vi "LCOS GUI v3_green.vi"() -> ()   [LabVIEW 2011]
uses:
  Periodic Spot Pattern Parameters.ctl
  LCOS State Machine States.ctl
  LCOS Pattern Display Actions.ctl
  LCOS Parent Action.ctl
  LCOS Images.ctl
  <vilib>/vision/Image Controls.llb/IMAQ Image.ctl
panel:
  in  "Enable Remote Control":bool=TRUE
  in  "Clear Error":bool
  in  "Ignore":bool
  out "Last Error":errorcluster
  in  "Loaded Pattern File:":bool
  out "File Path":path
  out "LCOS Pattern Preview":T1(plugin-control)
  in  "Buttons":T2={"Pattern"=enum."Computed", "Auto-Update LCOS"=TRUE, "Apply Correction"=FALSE, "Update LCOS"=FALSE, "Preview Pattern"=FALSE, "Auto-Preview"=TRUE}
  in  "Pattern Definition":T3={"X pitch"=24.0, "rotation"=0.0, "Center H"=0.0, "Center V"=0.0, "# Spots H"=4, "# Spots V"=12, "Spot size"=20.0, "ref_spot _dark"=FALSE, "Exact Phase Formula"=FALSE, "phase_wrap_pos"=FALSE, "Set Focus (mm)"=36.0, "phase_max"=3.0, "phase_factor"=82, "Steer LW"=1, "Steer vmax"=95, "phase_wrap_neg"=TRUE, "steer_horiz"=TRUE, "steer_pad"=10, "steer_only"=FALSE, "Wavelength"=5.32e-07, "Y pitch"=24.0, "python"=TRUE, "test_pattern"=FALSE, "grid"=TRUE, "dark_all"=FALSE, "Xm_str"="", "Ym_str"="", "ref_spot"=6, "stretch"=FALSE} {"ref_spot" min=0 max=500 step=1 format="%#.0f"; "Y pitch" min=0.0 max=100.0 format="%.2g"; "Wavelength" min=0.0 max=500.0 format="%^#.3e"; "steer_pad" min=0 max=500 step=1 format="%#.0f"; "Steer LW" max=500; "phase_max" min=0.0 max=500.0 format="%#.3f"; "Set Focus (mm)" min=0.0 max=500.0 format="%#.3g"; "Spot size" min=1.0 format="%.2g"; "# Spots V" min=1 step=1; "# Spots H" min=1 step=1; "Center V" format="%.2f"; "Center H" format="%.2f"; "rotation" min=-90.0 max=90.0 format="%.2g"; "X pitch" min=0.0 max=100.0 format="%.2g"}
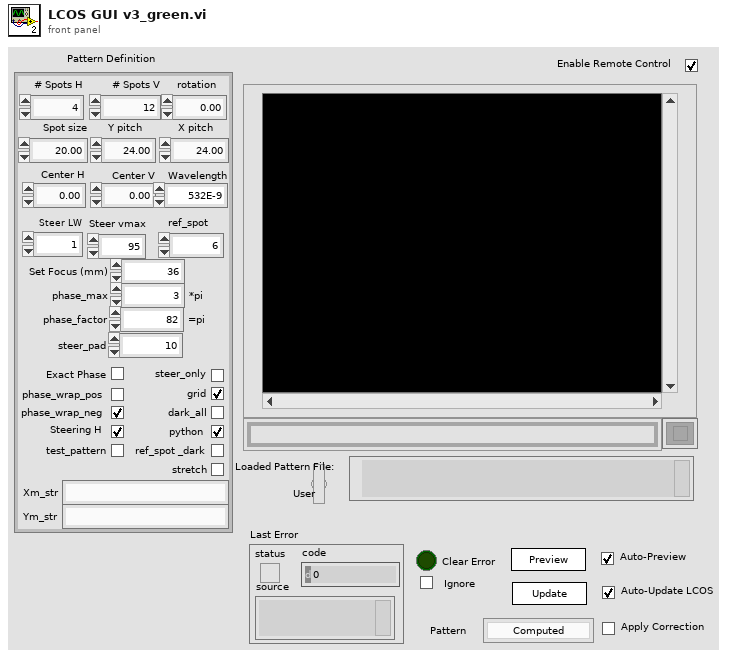
[diagram p1: front panel]
types:
  T1 = typedef "IMAQ Image.ctl" = refnum<image>
  T2 = cluster{"Pattern":enum16{"Computed", "From File", "Correction"}, "Auto-Update LCOS":bool, "Apply Correction":bool, "Update LCOS":bool, "Preview Pattern":bool, "Auto-Preview":bool}
  T3 = typedef "Periodic Spot Pattern Parameters.ctl" = cluster{"X pitch":dbl, "rotation":dbl, "Center H":dbl, "Center V":dbl, "# Spots H":u32, "# Spots V":u32, "Spot size":dbl, "ref_spot _dark":bool, "Exact Phase Formula":bool, "phase_wrap_pos":bool, "Set Focus (mm)":dbl, "phase_max":dbl, "phase_factor":u8, "Steer LW":u32, "Steer vmax":u8, "phase_wrap_neg":bool, "steer_horiz":bool, "steer_pad":i64, "steer_only":bool, "Wavelength":dbl, "Y pitch":dbl, "python":bool, "test_pattern":bool, "grid":bool, "dark_all":bool, "Xm_str":string, "Ym_str":string, "ref_spot":i64, "stretch":bool}
  T4 = typedef "LCOS Pattern Display Actions.ctl" = enum16{"Init", "Idle", "Update", "Exit"}
  T5 = cluster{"LCOS Pattern Display Actions":T4, "Data":variant}
  T6 = typedef "LCOS State Machine States.ctl" = enum16{"Init", "Idle", "Preview Button Pushed", "Update Button Pushed", "Pattern Selection Changed", "Pattern Definition Changed", "Selected File Changed", "Load Correction Pattern", "Load Correction Pattern Step 2", "Load User Pattern", "Load User Pattern Step 2", "Compute Pattern", "Correct Pattern", "Update Preview Display", "Update LCOS Display", "Error", "Clear Error", "Exit"}
  T7 = cluster{"X pitch":dbl, "rotation":dbl, "Center H":dbl, "Center V":dbl, "# Spots H":u32, "# Spots V":u32, "Spot size":dbl, "ref_spot _dark":bool, "Exact Phase Formula":bool, "phase_wrap_pos":bool, "Set Focus (mm)":dbl, "phase_max":dbl, "phase_factor":u8, "Steer LW":u32, "Steer vmax":u8, "phase_wrap_neg":bool, "steer_horiz":bool, "steer_pad":i64, "steer_only":bool, "Wavelength":dbl, "Y pitch":dbl, "python":bool, "test_pattern":bool, "grid":bool, "dark_all":bool, "Xm_str":string, "Ym_str":string, "ref_spot":i64, "stretch":bool}
  T8 = typedef "LCOS Parent Action.ctl" = enum16{"Pattern Definition Changed", "Preview Button Pushed", "Update Button Pushed", "Pattern Selection Changed", "Correction Pattern Changed", "User Pattern (from File) Changed"}
  T9 = typedef "LCOS Images.ctl" = cluster{"Computed Pattern Image":T1, "User Pattern (from File) Image":T1, "Correction Pattern Image":T1, "Corrected Pattern Image":T1, "Preview Image":T1, "LCOS Displayed Image":T1}
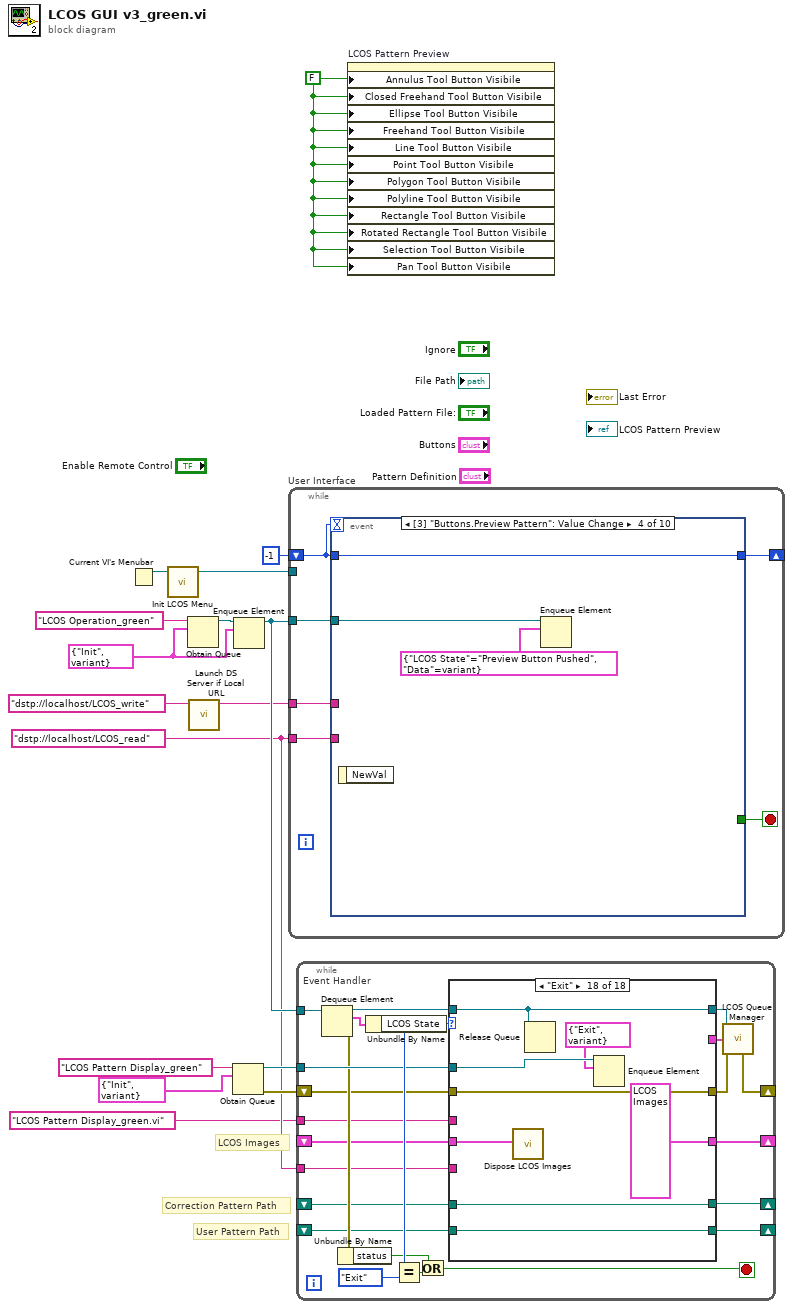
[diagram p0: block diagram]
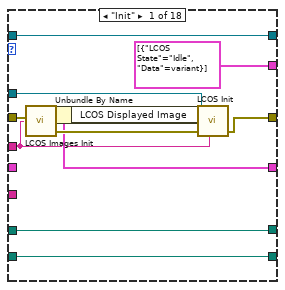
[diagram p2: hidden frame]
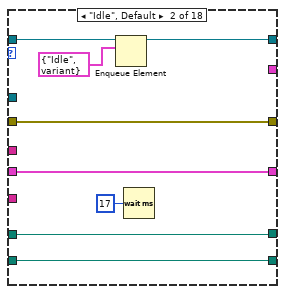
[diagram p3: hidden frame]
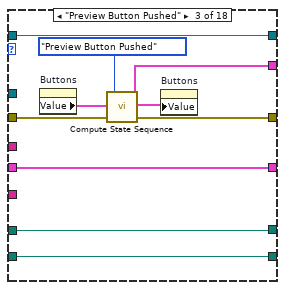
[diagram p4: hidden frame]
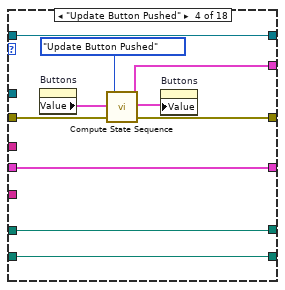
[diagram p5: hidden frame]
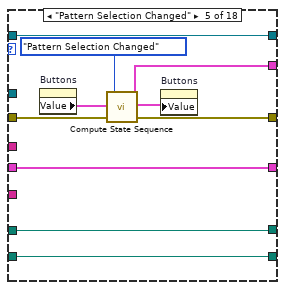
[diagram p6: hidden frame]
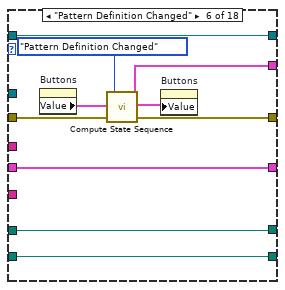
[diagram p7: hidden frame]
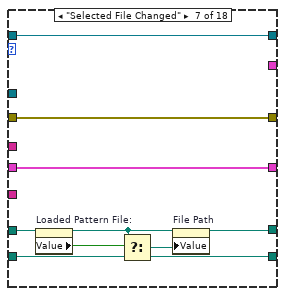
[diagram p8: hidden frame]
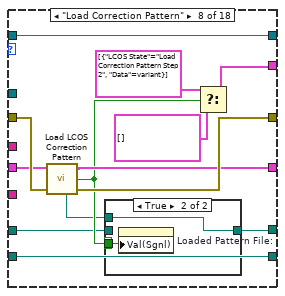
[diagram p9: hidden frame]
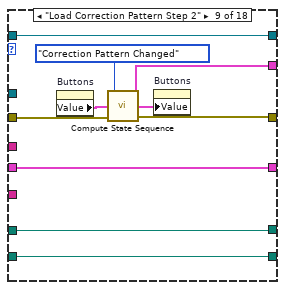
[diagram p11: hidden frame]
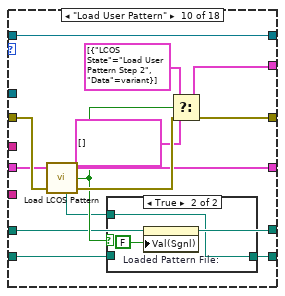
[diagram p12: hidden frame]
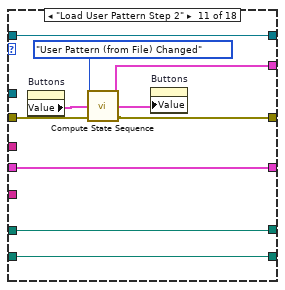
[diagram p14: hidden frame]
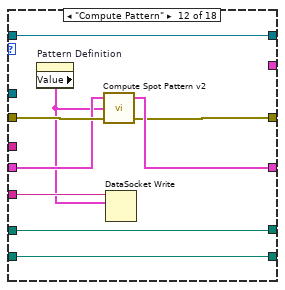
[diagram p15: hidden frame]
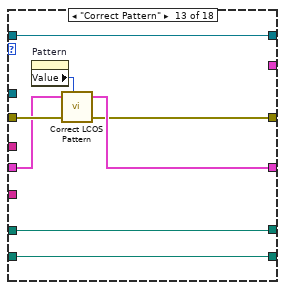
[diagram p16: hidden frame]
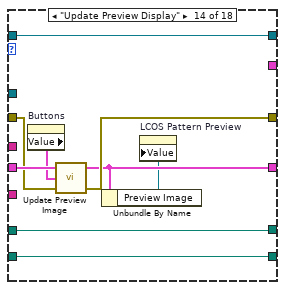
[diagram p17: hidden frame]
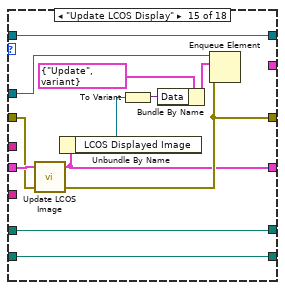
[diagram p18: hidden frame]
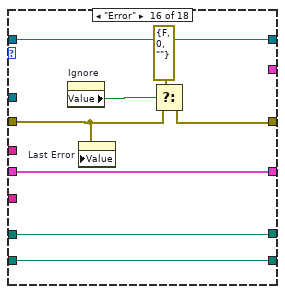
[diagram p19: hidden frame]
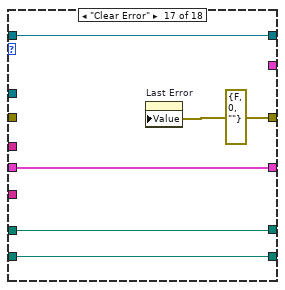
[diagram p20: hidden frame]
diagram:
  w2 = "dstp://localhost/LCOS_read" ("URL")
  w6 = FALSE ("ROI Tool Buttons Visibile:Annulus Tool Button Visibile")
  w7 = cluster{"LCOS State":T6, "Data":variant} {"LCOS State"=enum."Init", "Data"=variant}
  # "User Pattern Path"
  # "Correction Pattern Path"
  # "LCOS Images"
  n1 = Current VI's Menubar() -> (w16:refnum<k9>)
  n2 = call "Init LCOS Menu.vi"("Menu Refnum (in)"=w16) -> ("Menu Refnum (out)"=w15:refnum<k9>)  [unwired: 7 in, 1 out]
  n3 = Obtain Queue(name (unnamed)="LCOS Operation_green", element data type=w7) -> (queue out=w9:refnum<queue>)  [unwired: 3 in, 2 out]
  n4 = call "Launch DS Server if Local URL.vi"("URL"="dstp://localhost/LCOS_write") -> ("Duplicate URL"=w3:string)  [unwired: 5 in, 1 out]
  n5 = Obtain Queue(name (unnamed)="LCOS Pattern Display_green", element data type=T5 {"LCOS Pattern Display Actions"=enum."Init", "Data"=variant}) -> (queue out=w11:refnum<queue>, error out=w10:errorcluster)  [unwired: 3 in, 1 out]
  n6 = Enqueue Element(queue=w9, element=w7) -> (queue out=w8:refnum<queue>)  [unwired: 2 in, 2 out]
  n7 = while "User Interface" {
    tunnel: w15 -> [_]
    tunnel: w8 -> [w21]
    shift-right: [w20] -> _
    shift-left: -1 -> [w19]
    tunnel: w3 -> [w18]
    tunnel: w2 -> [w17]
    stop <- w22 stop-if-true
    n8 = event shown="[3] \"Buttons.Preview Pattern\": Value Change" {
      selector: _ -> [_ _ _ _ _ _ _ _ _ _]
      dyn-events: _ -> [_ _ _ _ _ _ _ _ _ _]
      timeout: w19 -> [_ _ _ _ _ _ _ _ _ _]
      tunnel: [_ _ _ _ _ _ _ _ w58 w76] -> w22
      tunnel: w21 -> [_ _ w41 w44 w47 w50 w53 w56 w59 w75]
      tunnel: [w23 w35 w39 w42 w45 w48 w51 w54 w57 w73] -> w20
      tunnel: w19 -> [w23 _ w39 w42 w45 w48 w51 w54 w57 w73]
      tunnel: w18 -> [w28 _ _ _ _ _ _ _ _ _]
      tunnel: w17 -> [w24 w32 _ _ _ _ _ _ _ _]
      event Timeout {
        n9 = event-data() -> ()  [unwired: 1 in, 1 out]
        n10 = DataSocket Read(9:w23, 10:T3 {"X pitch"=0.0, "rotation"=0.0, "Center H"=0.0, "Center V"=0.0, "# Spots H"=0, "# Spots V"=0, "Spot size"=0.0, "ref_spot _dark"=FALSE, "Exact Phase Formula"=FALSE, "phase_wrap_pos"=FALSE, "Set Focus (mm)"=0.0, "phase_max"=0.0, "phase_factor"=0, "Steer LW"=0, "Steer vmax"=0, "phase_wrap_neg"=FALSE, "steer_horiz"=FALSE, "steer_pad"=0, "steer_only"=FALSE, "Wavelength"=0.0, "Y pitch"=0.0, "python"=FALSE, "test_pattern"=FALSE, "grid"=FALSE, "dark_all"=FALSE, "Xm_str"="", "Ym_str"="", "ref_spot"=0, "stretch"=FALSE} ("Pattern Definition"), 11:w28) -> (1:w26:bool, 2:w25:T3)  [unwired: 2 in, 5 out]
        n11 = case shown="False" w26 {
          tunnel: w25 -> [w30 _]
          tunnel: w24 -> [w31 _]
          tunnel: w23 -> [w29 _]
          frame False {
            n12 = property on="Pattern Definition" class="Clust (strict)"("Val(Sgnl)"=w30) -> ()  [unwired: 2 in, 2 out]
            n13 = DataSocket Write(9:w29, 10:w30, 11:w31) -> ()  [unwired: 1 in, 3 out]
          }
          frame True {
          }
        }
      }
      event "Enable Remote Control": Value Change {
        n14 = event-data() -> ("NewVal"=w33:bool)  [unwired: 1 in]
        n15 = case shown="False" w33 {
          tunnel: w32 -> [_ w38]
          frame False {
          }
          frame True {
            n16 = property on="Pattern Definition" class="Clust (strict)"() -> ("Value"=w37:T7)  [unwired: 2 in, 2 out]
            n17 = DataSocket Write(10:w37, 11:w38) -> ()  [unwired: 2 in, 3 out]
          }
        }
        n18 = Select(t=1, s=w33, f=-1) -> (s? t:f=w35:i32)
      }
      event Value Change {
        n19 = event-data() -> ()  [unwired: 1 in, 1 out]
        n20 = Enqueue Element(queue=w41, element=cluster{"LCOS State":T6, "Data":variant} {"LCOS State"=enum."Pattern Definition Changed", "Data"=variant}) -> ()  [unwired: 2 in, 3 out]
      }
      event "Buttons.Preview Pattern": Value Change {
        n21 = event-data() -> ()  [unwired: 1 in, 1 out]
        n22 = Enqueue Element(queue=w44, element=cluster{"LCOS State":T6, "Data":variant} {"LCOS State"=enum."Preview Button Pushed", "Data"=variant}) -> ()  [unwired: 2 in, 3 out]
      }
      event "Buttons.Update LCOS": Value Change {
        n23 = event-data() -> ()  [unwired: 1 in, 1 out]
        n24 = Enqueue Element(queue=w47, element=cluster{"LCOS State":T6, "Data":variant} {"LCOS State"=enum."Update Button Pushed", "Data"=variant}) -> ()  [unwired: 2 in, 3 out]
      }
      event "Buttons.Pattern": Value Change {
        n25 = event-data() -> ()  [unwired: 1 in, 4 out]
        n26 = Enqueue Element(queue=w50, element=cluster{"LCOS State":T6, "Data":variant} {"LCOS State"=enum."Pattern Selection Changed", "Data"=variant}) -> ()  [unwired: 2 in, 3 out]
      }
      event "Clear Error": Value Change {
        n27 = event-data() -> ()  [unwired: 1 in, 1 out]
        n28 = Enqueue Element(queue=w53, element=cluster{"LCOS State":T6, "Data":variant} {"LCOS State"=enum."Clear Error", "Data"=variant}) -> ()  [unwired: 2 in, 3 out]
      }
      event "Loaded Pattern File:": Value Change {
        n29 = event-data() -> ()  [unwired: 1 in, 1 out]
        n30 = Enqueue Element(queue=w56, element=cluster{"LCOS State":T6, "Data":variant} {"LCOS State"=enum."Selected File Changed", "Data"=variant}) -> ()  [unwired: 2 in, 3 out]
      }
      event Menu Selection (User) {
        n31 = event-data() -> ("ItemTag"=w60:string)  [unwired: 1 in]
        n32 = case shown="\"Load Correction Pattern\"" w60 {
          tunnel: w59 -> [_ w62 w64 w68]
          tunnel: [_ _ _ w65] -> w58
          frame "-", Default {
          }
          frame "Load Correction Pattern" {
            n33 = Enqueue Element(queue=w62, element=cluster{"LCOS State":T6, "Data":variant} {"LCOS State"=enum."Load Correction Pattern", "Data"=variant}) -> ()  [unwired: 2 in, 3 out]
          }
          frame "Load User Pattern" {
            n34 = Enqueue Element(queue=w64, element=cluster{"LCOS State":T6, "Data":variant} {"LCOS State"=enum."Load User Pattern", "Data"=variant}) -> ()  [unwired: 2 in, 3 out]
          }
          frame "Quit" {
            n35 = Two Button Dialog(message="Do you want to quit?") -> (T button?=w65:bool)  [unwired: 2 in]
            n36 = case shown="True" w65 {
              tunnel: w68 -> [w69 w72]
              tunnel: [w69 w71] -> _
              tunnel: cluster{"LCOS State":T6, "Data":variant} {"LCOS State"=enum."Exit", "Data"=variant} ("element") -> [_ w70]
              frame False {
              }
              frame True {
                n37 = Enqueue Element(queue=w72, element=w70) -> (queue out=w71:refnum<queue>)  [unwired: 2 in, 2 out]
              }
            }
          }
        }
      }
      event Panel Close? {
        w76 = TRUE ("Discard?")
        n38 = event-data() -> ()  [unwired: 1 in, 1 out]
        n39 = Enqueue Element(queue=w75, element=cluster{"LCOS State":T6, "Data":variant} {"LCOS State"=enum."Exit", "Data"=variant}) -> ()  [unwired: 2 in, 3 out]
        n40 = event-data("Discard?"=w76) -> ()  [unwired: 1 in, 1 out]
      }
    }
  }
  n41 = while "Event Handler" {
    tunnel: w11 -> [w94]
    shift-right: [w88] -> _
    shift-left: w10 -> [w86]
    tunnel: w8 -> [w99]
    shift-right: [w84] -> _
    shift-left: _ -> [w85]
    shift-right: [w82] -> _
    shift-left: _ -> [w81]
    shift-right: [w80] -> _
    shift-left: _ -> [w79]
    tunnel: w2 -> [w78]
    tunnel: "LCOS Pattern Display_green.vi" ("name (unnamed)") -> [w77]
    stop <- w91 stop-if-true
    n42 = Dequeue Element(queue=w99) -> (queue out=w95:refnum<queue>, element=w93:cluster{"LCOS State":T6, "Data":variant}, error out=w92:errorcluster)  [unwired: 2 in, 1 out]
    n43 = Unbundle By Name(w92) -> ("status"=w90:bool)
    n44 = Unbundle By Name(w93) -> ("LCOS State"=w98:T6)
    n45 = Equal?(x=w98, y=LCOS_State_Machine_States."Exit") -> (x = y?=w96:bool)
    n46 = Or(x=w90, y=w96) -> (x .or. y?=w91:bool)
    n47 = case shown="\"Exit\"" w98 {
      tunnel: w95 -> [w103 w118 w125 w135 w145 w155 w165 w173 w189 w199 w215 w222 w229 w243 w251 w258 w266 w271]
      tunnel: w94 -> [w110 _ _ _ _ _ _ _ _ _ _ _ _ _ w255 _ _ w275]
      tunnel: [cluster{"LCOS State":T6, "Data":variant}[] [{"LCOS State"=enum."Idle", "Data"=variant}] ("Action Sequence") _ w122 w132 w142 w152 _ w176 w186 w201 w212 _ _ _ _ _ _ _] -> w89
      tunnel: [w109 w116 w123 w133 w143 w153 w164 w177 w187 w203 w213 w223 w230 w239 w248 w261 w268 w276] -> w87
      tunnel: w86 -> [w108 w116 w124 w134 w144 w154 w164 w178 w188 w204 w214 w226 w233 w240 w249 w259 _ w276]
      tunnel: w85 -> [_ w114 w127 w137 w147 w157 w163 w172 w184 w198 w210 w225 w232 w242 w250 w263 w267 w273]
      tunnel: [w105 w114 w127 w137 w147 w157 w163 w171 w184 w197 w210 w224 w231 w238 w247 w263 w267 T9 {"Computed Pattern Image"=refnum, "User Pattern (from File) Image"=refnum, "Correction Pattern Image"=refnum, "Corrected Pattern Image"=refnum, "Preview Image"=refnum, "LCOS Displayed Image"=refnum} ("Images")] -> w84
      tunnel: [w103 w113 w125 w135 w145 w155 w165 w173 w189 w199 w215 w222 w229 w243 w251 w258 w266 w271] -> w83
      tunnel: [w102 w112 w120 w130 w140 w150 w160 w168 w183 w192 w209 w221 w228 w236 w245 w257 w265 w270] -> w82
      tunnel: w81 -> [w102 w112 w120 w130 w140 w150 w160 w169 w183 w192 w209 w221 w228 w236 w245 w257 w265 w270]
      tunnel: [w101 w111 w119 w129 w139 w149 w161 w166 w182 w194 w208 w220 w227 w235 w244 w256 w264 w269] -> w80
      tunnel: w79 -> [w101 w111 w119 w129 w139 w149 w161 w166 w182 w193 w208 w220 w227 w235 w244 w256 w264 w269]
      tunnel: w78 -> [_ _ _ _ _ _ _ _ _ _ _ w219 _ _ _ _ _ _]
      tunnel: w77 -> [w100 _ _ _ _ _ _ _ _ _ _ _ _ _ _ _ _ _]
      frame "Init" {
        n48 = call "LCOS Images Init.vi"("LCOS Pattern Display.vi Name"=w100, "error in (no error)"=w108) -> ("Images"=w105:T9, "error out"=w107:errorcluster)  [unwired: 6 in]
        n49 = Unbundle By Name(w105) -> ("LCOS Displayed Image"=w106:T1)
        n50 = call "LCOS Init.vi"("LCOS Display Queue"=w110, "LCOS Displayed Image"=w106, "error in (no error)"=w107, "LCOS Pattern Display.vi Name"=w100) -> ("error out"=w109:errorcluster)  [unwired: 5 in]
      }
      frame "Idle", Default {
        n51 = Enqueue Element(queue=w118, element=cluster{"LCOS State":T6, "Data":variant} {"LCOS State"=enum."Idle", "Data"=variant}) -> (queue out=w113:refnum<queue>)  [unwired: 2 in, 2 out]
        n52 = Wait (ms)(milliseconds to wait=u32 17) -> ()  [unwired: 1 out]
      }
      frame "Preview Button Pushed" {
        n53 = property on="Buttons" class="Clust (strict)"() -> ("Value"=w128:T2)  [unwired: 2 in, 2 out]
        n54 = call "Compute State Sequence.vi"("Parent Action"=LCOS_Parent_Action."Preview Button Pushed" ("Previous Event"), "Buttons (in)"=w128, "error in (no error)"=w124) -> ("Action Sequence"=w122:cluster{"LCOS State":T6, "Data":variant}[], "Buttons (out)"=w121:T2, "error out"=w123:errorcluster)  [unwired: 4 in]
        n55 = property on="Buttons" class="Clust (strict)"("Value"=w121) -> ()  [unwired: 2 in, 2 out]
      }
      frame "Update Button Pushed" {
        n56 = property on="Buttons" class="Clust (strict)"() -> ("Value"=w138:T2)  [unwired: 2 in, 2 out]
        n57 = call "Compute State Sequence.vi"("Parent Action"=LCOS_Parent_Action."Update Button Pushed" ("Previous Event"), "Buttons (in)"=w138, "error in (no error)"=w134) -> ("Action Sequence"=w132:cluster{"LCOS State":T6, "Data":variant}[], "Buttons (out)"=w131:T2, "error out"=w133:errorcluster)  [unwired: 4 in]
        n58 = property on="Buttons" class="Clust (strict)"("Value"=w131) -> ()  [unwired: 2 in, 2 out]
      }
      frame "Pattern Selection Changed" {
        n59 = property on="Buttons" class="Clust (strict)"() -> ("Value"=w148:T2)  [unwired: 2 in, 2 out]
        n60 = call "Compute State Sequence.vi"("Parent Action"=LCOS_Parent_Action."Pattern Selection Changed" ("Previous Event"), "Buttons (in)"=w148, "error in (no error)"=w144) -> ("Action Sequence"=w142:cluster{"LCOS State":T6, "Data":variant}[], "Buttons (out)"=w141:T2, "error out"=w143:errorcluster)  [unwired: 4 in]
        n61 = property on="Buttons" class="Clust (strict)"("Value"=w141) -> ()  [unwired: 2 in, 2 out]
      }
      frame "Pattern Definition Changed" {
        n62 = property on="Buttons" class="Clust (strict)"() -> ("Value"=w158:T2)  [unwired: 2 in, 2 out]
        n63 = call "Compute State Sequence.vi"("Parent Action"=LCOS_Parent_Action."Pattern Definition Changed" ("Previous Event"), "Buttons (in)"=w158, "error in (no error)"=w154) -> ("Action Sequence"=w152:cluster{"LCOS State":T6, "Data":variant}[], "Buttons (out)"=w151:T2, "error out"=w153:errorcluster)  [unwired: 4 in]
        n64 = property on="Buttons" class="Clust (strict)"("Value"=w151) -> ()  [unwired: 2 in, 2 out]
      }
      frame "Selected File Changed" {
        n65 = property on="Loaded Pattern File:" class="Bool (strict)"() -> ("Value"=w162:bool)  [unwired: 2 in, 2 out]
        n66 = Select(t=w160, s=w162, f=w161) -> (s? t:f=w159:path)
        n67 = property on="File Path" class="Path"("Value"=w159) -> ()  [unwired: 2 in, 2 out]
      }
      frame "Load Correction Pattern" {
        n68 = call "Load LCOS Correction Pattern.vi"("Images Dest"=w172, "error in"=w178) -> ("Images Out"=w171:T9, "Correct File Type"=w170:bool, "Path"=w167:path, "error out"=w177:errorcluster)  [unwired: 3 in, 1 out]
        n69 = case shown="True" w170 {
          tunnel: w170 -> [_ w181]
          tunnel: w169 -> [w179 _]
          tunnel: [w179 w180] -> w168
          tunnel: w167 -> [_ w180]
          frame False {
          }
          frame True {
            n70 = property on="Loaded Pattern File:" class="Bool (strict)"("Val(Sgnl)"=w181) -> ()  [unwired: 2 in, 2 out]
          }
        }
        n71 = Select(t=cluster{"LCOS State":T6, "Data":variant}[] [{"LCOS State"=enum."Load Correction Pattern Step 2", "Data"=variant}], s=w170, f=cluster{"LCOS State":T6, "Data":variant}[] []) -> (s? t:f=w176:cluster{"LCOS State":T6, "Data":variant}[])
      }
      frame "Load Correction Pattern Step 2" {
        n72 = property on="Buttons" class="Clust (strict)"() -> ("Value"=w191:T2)  [unwired: 2 in, 2 out]
        n73 = call "Compute State Sequence.vi"("Parent Action"=LCOS_Parent_Action."Correction Pattern Changed" ("Previous Event"), "Buttons (in)"=w191, "error in (no error)"=w188) -> ("Action Sequence"=w186:cluster{"LCOS State":T6, "Data":variant}[], "Buttons (out)"=w185:T2, "error out"=w187:errorcluster)  [unwired: 4 in]
        n74 = property on="Buttons" class="Clust (strict)"("Value"=w185) -> ()  [unwired: 2 in, 2 out]
      }
      frame "Load User Pattern" {
        n75 = call "Load LCOS Pattern.vi"("Images Dest"=w198, "error in"=w204) -> ("Images Out"=w197:T9, "Correct File Type"=w196:bool, "Path"=w195:path, "error out"=w203:errorcluster)  [unwired: 3 in, 1 out]
        n76 = case shown="True" w196 {
          tunnel: w193 -> [w205 _]
          tunnel: [w205 w207] -> w194
          tunnel: w195 -> [_ w207]
          frame False {
          }
          frame True {
            n77 = property on="Loaded Pattern File:" class="Bool (strict)"("Val(Sgnl)"=FALSE ("Value (Signaling)")) -> ()  [unwired: 2 in, 2 out]
          }
        }
        n78 = Select(t=cluster{"LCOS State":T6, "Data":variant}[] [{"LCOS State"=enum."Load User Pattern Step 2", "Data"=variant}], s=w196, f=cluster{"LCOS State":T6, "Data":variant}[] []) -> (s? t:f=w201:cluster{"LCOS State":T6, "Data":variant}[])
      }
      frame "Load User Pattern Step 2" {
        n79 = property on="Buttons" class="Clust (strict)"() -> ("Value"=w217:T2)  [unwired: 2 in, 2 out]
        n80 = call "Compute State Sequence.vi"("Parent Action"=LCOS_Parent_Action."User Pattern (from File) Changed" ("Previous Event"), "Buttons (in)"=w217, "error in (no error)"=w214) -> ("Action Sequence"=w212:cluster{"LCOS State":T6, "Data":variant}[], "Buttons (out)"=w211:T2, "error out"=w213:errorcluster)  [unwired: 4 in]
        n81 = property on="Buttons" class="Clust (strict)"("Value"=w211) -> ()  [unwired: 2 in, 2 out]
      }
      frame "Compute Pattern" {
        n82 = property on="Pattern Definition" class="Clust (strict)"() -> ("Value"=w218:T7)  [unwired: 2 in, 2 out]
        n83 = call "Compute Spot Pattern v2.vi"("Images Dest"=w225, "Pattern Definition"=w218, "error in"=w226) -> ("Images Out"=w224:T9, "error out"=w223:errorcluster)  [unwired: 3 in, 2 out]
        n84 = DataSocket Write(10:w218, 11:w219) -> ()  [unwired: 2 in, 3 out]
      }
      frame "Correct Pattern" {
        n85 = property on="Pattern" class="Enum (strict)"() -> ("Value"=w234:enum16{"Computed", "From File", "Correction"})  [unwired: 2 in, 2 out]
        n86 = call "Correct LCOS Pattern.vi"("Images Dest"=w232, "Pattern"=w234, "error in"=w233) -> ("Images Out"=w231:T9, "error out"=w230:errorcluster)  [unwired: 5 in]
      }
      frame "Update Preview Display" {
        n87 = property on="Buttons" class="Clust (strict)"() -> ("Value"=w241:T2)  [unwired: 2 in, 2 out]
        n88 = call "Update Preview Image.vi"("Images (Dest)"=w242, "Buttons"=w241, "error in"=w240) -> ("Images (Out)"=w238:T9, "error out"=w239:errorcluster)  [unwired: 5 in]
        n89 = Unbundle By Name(w238) -> ("Preview Image"=w237:T1)
        n90 = property on="LCOS Pattern Preview" class="ImageControl"("Value"=w237) -> ()  [unwired: 2 in, 2 out]
      }
      frame "Update LCOS Display" {
        n91 = call "Update LCOS Image.vi"("Images (Dest)"=w250, "error in"=w249) -> ("Images (Out)"=w247:T9, "error out"=w248:errorcluster)  [unwired: 6 in]
        n92 = Unbundle By Name(w247) -> ("LCOS Displayed Image"=w246:T1)
        n93 = To Variant(anything=w246) -> (Variant=w252:variant)
        n94 = Bundle By Name(cluster=T5 {"LCOS Pattern Display Actions"=enum."Update", "Data"=variant}, "Data"=w252) -> (w253:T5)
        n95 = Enqueue Element(queue=w255, element=w253, error in (no error)=w248) -> ()  [unwired: 1 in, 3 out]
      }
      frame "Error" {
        n96 = property on="Ignore" class="Bool (strict)"() -> ("Value"=w262:bool)  [unwired: 2 in, 2 out]
        n97 = property on="Last Error" class="Clust (strict)"("Value"=w259) -> ()  [unwired: 2 in, 2 out]
        n98 = Select(t=errorcluster {"status"=FALSE, "code"=0, "source"=""}, s=w262, f=w259) -> (s? t:f=w261:errorcluster)
      }
      frame "Clear Error" {
        w268 = errorcluster {"status"=FALSE, "code"=0, "source"=""} ("error out")
        n99 = property on="Last Error" class="Clust (strict)"("Value"=w268) -> ()  [unwired: 2 in, 2 out]
      }
      frame "Exit" {
        n100 = call "Dispose LCOS Images.vi"("Images"=w273) -> ()
        n101 = Release Queue(queue=w271) -> ()  [unwired: 2 in, 3 out]
        n102 = Enqueue Element(queue=w275, element=T5 {"LCOS Pattern Display Actions"=enum."Exit", "Data"=variant}) -> ()  [unwired: 2 in, 3 out]
      }
    }
    n103 = call "LCOS Queue Manager.vi"("Queue"=w83, "Queue States"=w89, "error in (no error)"=w87) -> ("error out"=w88:errorcluster)  [unwired: 6 in]
  }
  n104 = property on="LCOS Pattern Preview" class="ImageControl"("Annulus Tool Button Visibile"=w6, "Closed Freehand Tool Button Visibile"=w6, "Ellipse Tool Button Visibile"=w6, "Freehand Tool Button Visibile"=w6, "Line Tool Button Visibile"=w6, "Point Tool Button Visibile"=w6, "Polygon Tool Button Visibile"=w6, "Polyline Tool Button Visibile"=w6, "Rectangle Tool Button Visibile"=w6, "Rotated Rectangle Tool Button Visibile"=w6, "Selection Tool Button Visibile"=w6, "Pan Tool Button Visibile"=w6) -> ()  [unwired: 2 in, 2 out]
